vi "Send Update Generation On Fly Msg.vi"(8 "error in":errorcluster, 10 "signal settings":T1, 11 "Qbus in":refnum<class "Qbus.lvclass">) -> (0 "error out":errorcluster, 3 "Qbus out":refnum<class "Qbus.lvclass">)   [LabVIEW 2021, in "DigitalAudioGenerationProcess.lvlib"]
uses:
  DigitalAudioGenerationProcess.lvlib
  <vilib>/addons/Qbus/Qbus.lvclass
  controls/signal type.ctl
  controls/AudioGenTypeDefs.lvlib
  controls/signal settings.ctl
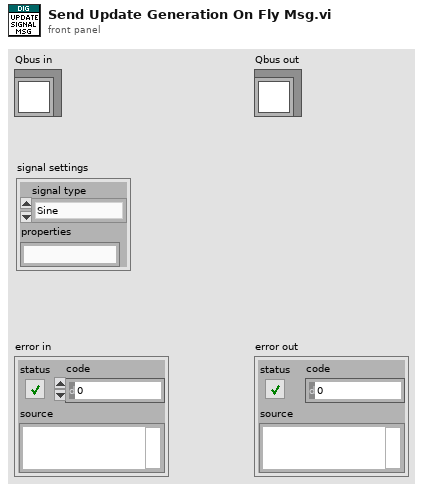
[diagram p1: front panel]
types:
  T1 = typedef "AudioGenTypeDefs.lvlib/signal settings.ctl" = cluster{"signal type":T2, "properties":string}
  T2 = typedef "AudioGenTypeDefs.lvlib/signal type.ctl" = enum16{"Sine", "Square", "Triangle", "White Noise", "Pink Noise", "Periodic Random Noise"}
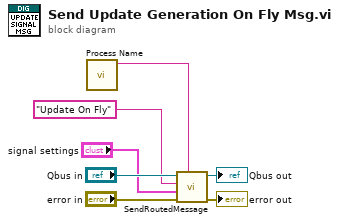
[diagram p0: block diagram]
diagram:
  n1 = call "Process Name.vi"() -> ("process name"=w2:string)  [unwired: 11 in]
  n2 = call <vilib>:"SendRoutedMessage.vi"("listener process"=w2, "error in (no error)"="error in", "message value"="signal settings", "message name"="Update On Fly", "Qbus in"="Qbus in") -> ("error in (no error)"=→"error out":errorcluster, "Qbus out"=→"Qbus out":refnum<class "Qbus.lvclass">)  [unwired: 5 in]
